vi "Durability_will_2012_07_04_motor not running.vi"() -> ()   [LabVIEW 2011]
uses:
  <vilib>/DAQmx/write.llb/DAQmx Write (Counter Time 1Chan 1Samp).vi
  <vilib>/DAQmx/read.llb/DAQmx Read (Analog 1D Wfm NChan NSamp).vi
  <vilib>/express/express shared/ex_Modify Signal Name.vi
  <vilib>/measure/madcrms.llb/Basic Averaged DC-RMS for 1 Chan.vi
  <vilib>/DAQmx/miscellaneous.llb/DAQmx Fill In Error Info.vi
  <vilib>/measure/madcrms.llb/Averaged DC-RMS for N Chan.vi
  <vilib>/express/express arith-compare/Formula/XNode/ExpressFormulaBlockNode.xnode
  <vilib>/measure/NI_MAPro.lvlib
panel:
  out "Collected Signals":dbl
  out "Table":string[][](table)
  in  "Filename 2":path=path "\\\\vmware-host\\Shared Folders/Desktop/long.tdms" caption="Filename"
  in  "Filename":path=path "\\\\vmware-host\\Shared Folders/Desktop/short.tdms"
  out "RPM Graph":dbl(graph)
  out "Motor RPM":dbl format="%#.0f"
  out "Motor Power (watts)":dbl format="%#.4f"
  out "Power to MC1 (watts)":dbl format="%#.4f"
  out "Voltage to MC1 (volts)":dbl format="%#.4f"
  out "Current to MC1  (amps)":dbl format="%#.4f"
  in  "Manual Start":bool
  in  "Power \nSetting":i8(slide) min=0 max=100 step=10 scale=0.0..100.0
  out "Power Setting (%)":dbl format="%#.2f"
  out "Motor Temp (F)":dbl format="%.1f"
  out "Tank Temp (F)":dbl format="%.1f"
  in  "Quit 4":bool
  out "Motor Power Over Time":dbl(graph)
  out "Phase to Phase Voltage":waveform(dbl)(graph)
  out "Phase Current":waveform(dbl)(graph)
  # "Motor Power and RPM"
  # "Temperature"
  # "MC1"
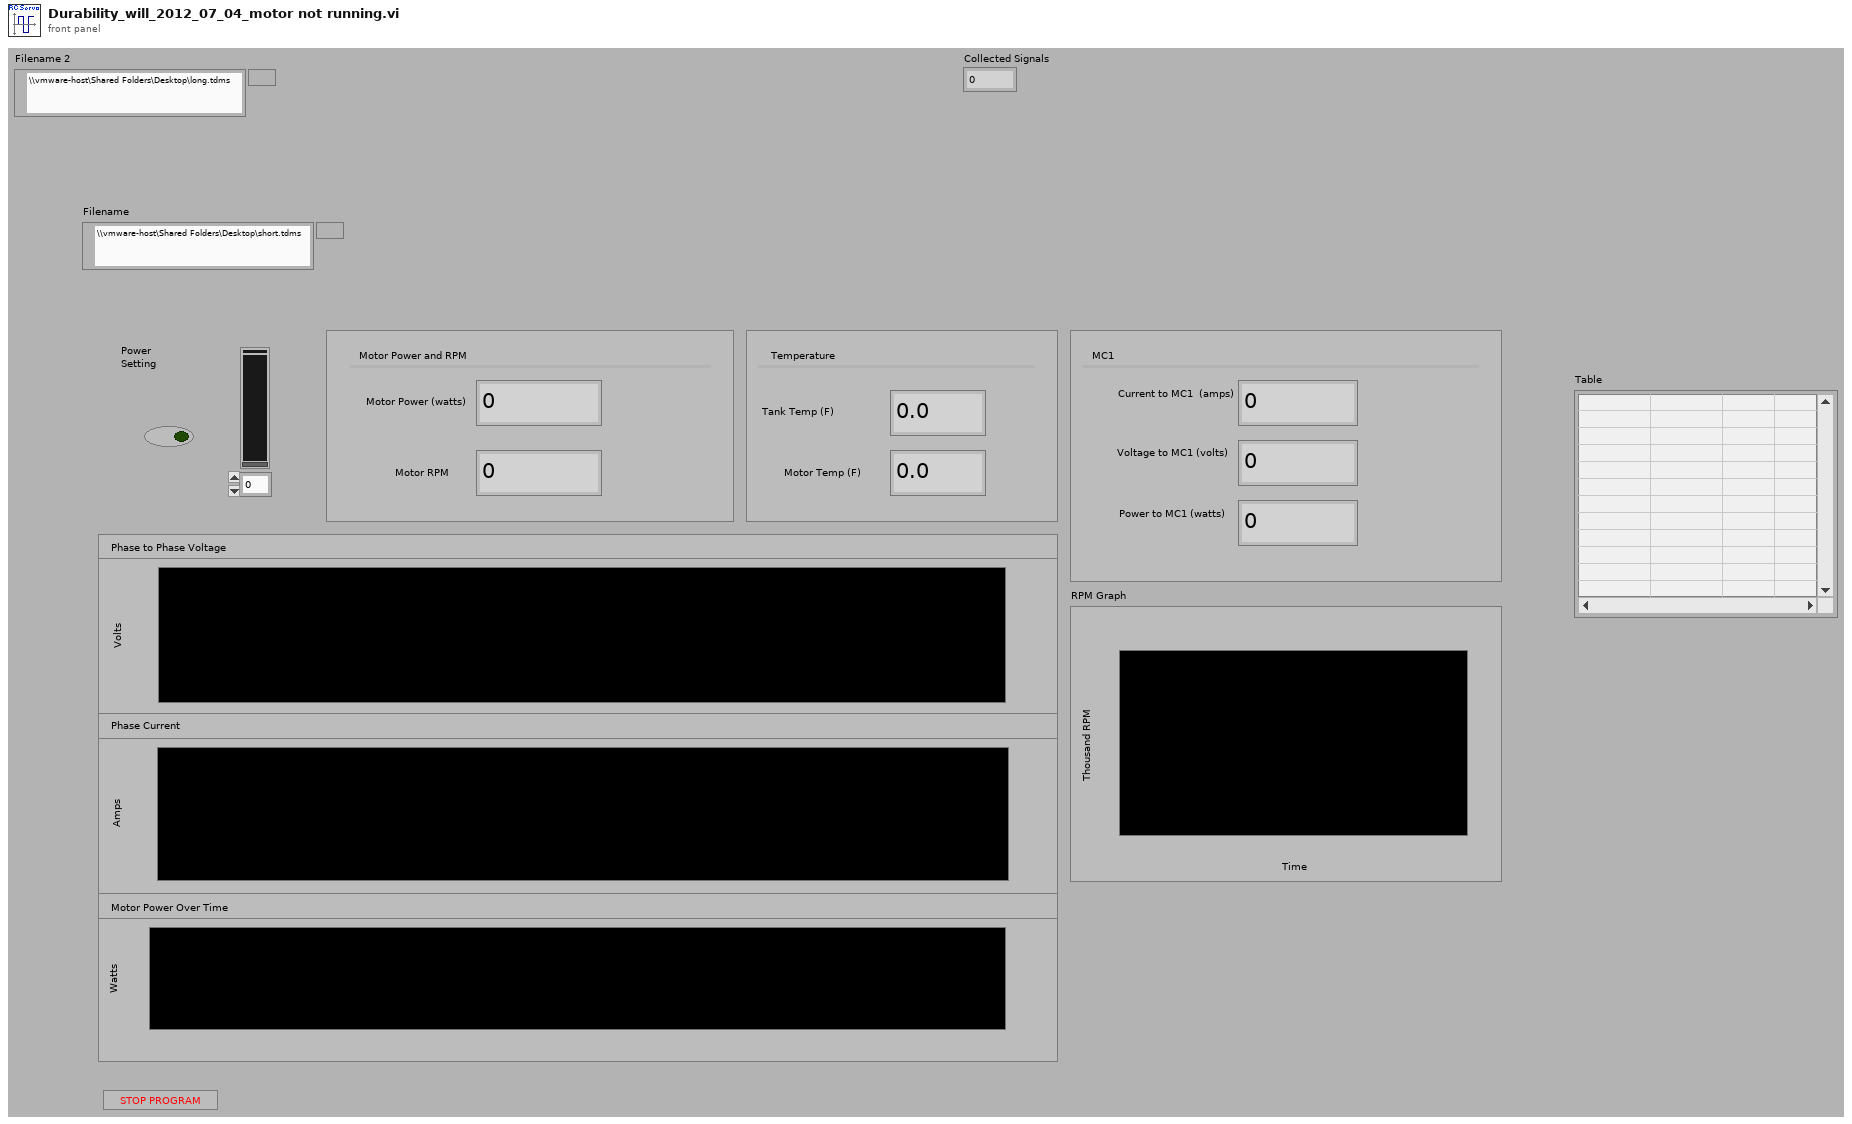
[diagram p1: front panel]
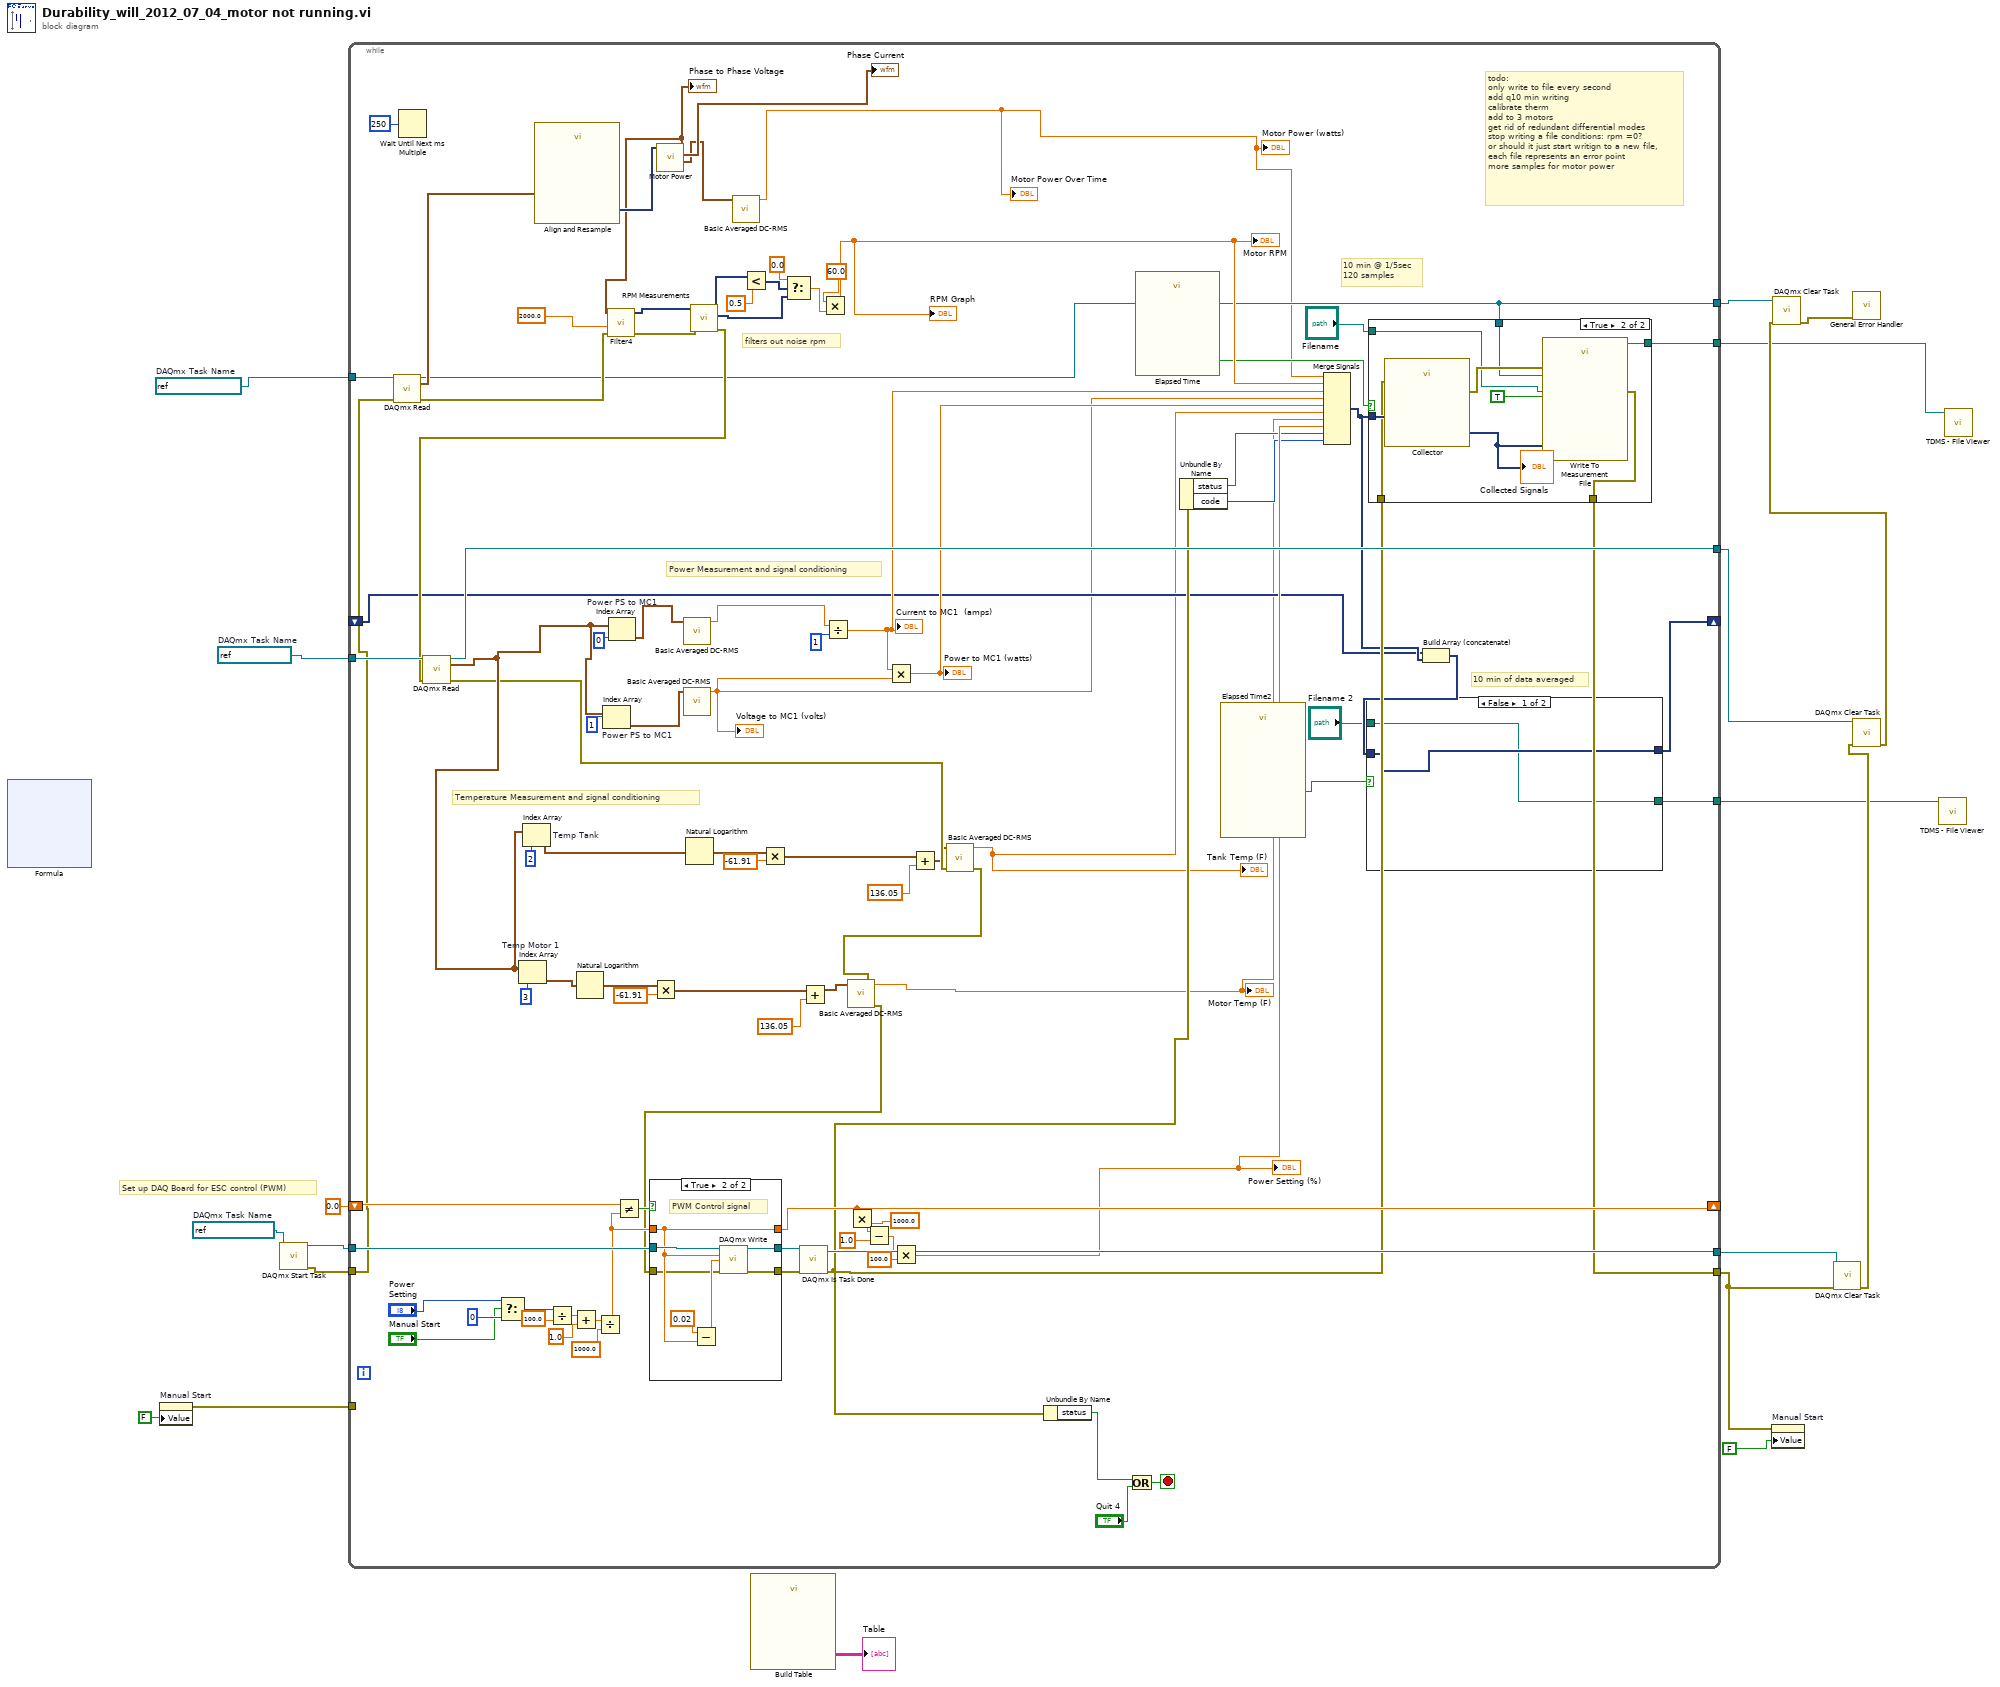
[diagram p0: block diagram]
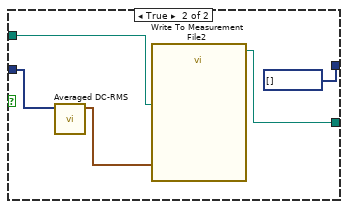
[diagram p2: hidden frame]
diagram:
  w10 = refnum<k21> "PWM Signal"  # DAQmx Task Name
  w15 = refnum<k21> "MC Power"  # DAQmx Task Name
  w16 = refnum<k21> "Motor Power"  # DAQmx Task Name
  # "Set up DAQ Board for ESC control (PWM)"
  n1 = xnode "Formula"() -> ()  [unwired: 2 in, 2 out]
  n2 = property on="Manual Start" class="Bool (strict)"("Value"=FALSE ("Run Motor")) -> (error out=w13:errorcluster)  [unwired: 2 in, 1 out]
  n3 = call <vilib>:"DAQmx Start Task.vi"("task/channels in"=w10) -> ("task out"=w9:refnum<k21>, "error out"=w8:errorcluster)  [unwired: 13 in]
  n4 = while {
    tunnel: [w113] -> w19
    tunnel: [w46] -> w11
    tunnel: w9 -> [w111]
    shift-right: [w94] -> _
    shift-left: 0.0 -> [w102]
    tunnel: w15 -> [w89]
    tunnel: [w88] -> w18
    tunnel: [w45] -> w17
    tunnel: w16 -> [w75]
    tunnel: w13 -> [_]
    tunnel: w8 -> [w68]
    shift-right: [w39] -> _
    shift-left: _ -> [w41]
    tunnel: [w38] -> w4
    tunnel: [w35] -> w3
    stop <- w71 stop-if-true
    # "10 min of data averaged"
    # "todo:\nonly write to file every second\nadd q10 min writing\ncalibrate therm\nadd to 3 motors\nget rid of redundant differential modes\nstop writing a file conditions: rpm =0?\nor should it just start writign to a new file,\neach file represents an error point\nmore samples for motor power"
    # "filters out noise rpm"
    # "10 min @ 1/5sec\n120 samples"
    # "Power Measurement and signal conditioning"
    # "Temperature Measurement and signal conditioning"
    n5 = call-poly <vilib>:"DAQmx Read.vi"("task/channels in"=w75, "error in"=w68) -> ("task out"=w45:refnum<k21>, "data"=w50:waveform(dbl)[], "error out"=w85:errorcluster)  [unwired: 11 in]
    n6 = Wait Until Next ms Multiple(millisecond multiple=u32 250) -> ()  [unwired: 1 out]
    n7 = Select(t="Power \nSetting", s="Manual Start", f=i8 0) -> (s? t:f=w100:i8)
    n8 = call "Align and Resample"("Signals"=w50) -> ("Resampled Signals"=w51:dynamicdata)  [unwired: 8 in, 2 out]
    n9 = Divide(x=w100, y=100.0) -> (x/y=w106:dbl)
    n10 = Add(x=w106, y=1.0 ("x/y")) -> (x+y=w104:dbl)
    n11 = Divide(x=w104, y=1000.0) -> (x/y=w103:dbl)
    n12 = Not Equal?(x=w102, y=w103) -> (x != y?=w112:bool)
    n13 = call "Motor Power.vi"("data"=w51) -> ("Waveform"=w34:waveform(dbl), "Phase Current"=→"Phase Current":waveform(dbl), "Phase to Phase Voltage"=w48:waveform(dbl))  [unwired: 7 in, 1 out]
    "Phase to Phase Voltage" <- w48
    n14 = call "Filter4"("error in (no error)"=w85, "Lower Cut-Off"=2000.0 ("LowPass Filter CutOff [Hz]"), "Signal"=w48) -> ("error out"=w86:errorcluster, "Filtered Signal"=w77:dynamicdata)  [unwired: 7 in]
    n15 = call "RPM Measurements"("error in (no error)"=w86, "Signals"=w77) -> ("error out"=w70:errorcluster, "Frequency"=w81:dynamicdata, "Amplitude"=w78:dynamicdata)  [unwired: 7 in]
    n16 = call-poly <vilib>:"DAQmx Read.vi"("task/channels in"=w89, "error in"=w70) -> ("task out"=w88:refnum<k21>, "data"=w27:waveform(dbl)[], "error out"=w25:errorcluster)  [unwired: 11 in]
    n17 = Index Array "Temp Motor 1"(array=w27, index=3) -> (element=w63:waveform(dbl))
    n18 = Index Array "Temp Tank"(array=w27, index=2) -> (element=w28:waveform(dbl))
    n19 = Natural Logarithm(1:w63) -> (0:w67:waveform(dbl))
    n20 = Index Array "Power PS to MC1"(array=w27, index=1) -> (element=w30:waveform(dbl))
    n21 = Index Array "Power PS to MC1"(array=w27, index=0) -> (element=w32:waveform(dbl))
    n22 = Multiply(x=w67, y=-61.91) -> (x*y=w65:waveform(dbl))
    n23 = call-poly <vilib>:"Basic Averaged DC-RMS.vi"("signal in"=w32) -> ("DC value"=w31:dbl)  [unwired: 7 in, 3 out]
    n24 = call-poly <vilib>:"Basic Averaged DC-RMS.vi"("signal in"=w30) -> ("DC value"=w29:dbl)  [unwired: 7 in, 3 out]
    "Voltage to MC1 (volts)" <- w29
    n25 = Natural Logarithm(1:w28) -> (0:w62:waveform(dbl))
    n26 = call-poly <vilib>:"Basic Averaged DC-RMS.vi"("signal in"=w34) -> ("DC value"=w33:dbl)  [unwired: 7 in, 3 out]
    "Motor Power Over Time" <- w33
    "Motor Power (watts)" <- w33
    n27 = Less?(x=w78, y=0.5) -> (x < y?=w80:dynamicdata)
    n28 = Multiply(x=w62, y=-61.91) -> (x*y=w60:waveform(dbl))
    n29 = Select(t=0.0, s=w80, f=w81) -> (s? t:f=w83:dbl)
    n30 = Add(x=w65, y=136.05) -> (x+y=w23:waveform(dbl))
    n31 = Multiply(x=60.0, y=w83) -> (x*y=w57:dbl)
    "Motor RPM" <- w57
    "RPM Graph" <- w57
    n32 = Divide(x=w31, y=1) -> (x/y=w56:dbl)
    "Current to MC1  (amps)" <- w56
    n33 = Multiply(x=w56, y=w29) -> (x*y=w55:dbl)
    "Power to MC1 (watts)" <- w55
    n34 = Add(x=w60, y=136.05) -> (x+y=w24:waveform(dbl))
    n35 = call-poly <vilib>:"Basic Averaged DC-RMS.vi"("error in (no error)"=w25, "signal in"=w24) -> ("error out"=w20:errorcluster, "DC value"=w26:dbl)  [unwired: 6 in, 2 out]
    "Tank Temp (F)" <- w26
    n36 = call-poly <vilib>:"Basic Averaged DC-RMS.vi"("error in (no error)"=w20, "signal in"=w23) -> ("error out"=w21:errorcluster, "DC value"=w22:dbl)  [unwired: 6 in, 2 out]
    "Motor Temp (F)" <- w22
    n37 = case shown="True" w112 {
      tunnel: w103 -> [w133 w136]
      tunnel: w111 -> [w134 w140]
      tunnel: [w134 w138] -> w110
      tunnel: [w132 w137] -> w109
      tunnel: [w133 w136] -> w94
      tunnel: w21 -> [w132 w135]
      frame False {
      }
      frame True {
        # "PWM Control signal"
        n38 = Subtract(x=0.02, y=w136) -> (x-y=w139:dbl)
        n39 = call-poly <vilib>:"DAQmx Write.vi"("task/channels in"=w140, "high time"=w136, "low time"=w139, "error in"=w135) -> ("task out"=w138:refnum<k21>, "error out"=w137:errorcluster)  [unwired: 9 in, 1 out]
      }
    }
    n40 = call <vilib>:"DAQmx Is Task Done.vi"("task/channels in"=w110, "error in"=w109) -> ("task out"=w113:refnum<k21>, "error out"=w47:errorcluster)  [unwired: 11 in, 1 out]
    n41 = Multiply(x=w94, y=1000.0) -> (x*y=w95:dbl)
    n42 = Subtract(x=w95, y=1.0) -> (x-y=w98:dbl)
    n43 = Multiply(x=w98, y=100.0) -> (x*y=w54:dbl)
    "Power Setting (%)" <- w54
    n44 = Unbundle By Name(w47) -> ("status"=w69:bool)
    n45 = Or(x=w69, y="Quit 4") -> (x .or. y?=w71:bool)
    n46 = call "Elapsed Time"() -> ("Time has Elapsed"=w44:bool)  [unwired: 12 in, 7 out]
    n47 = Unbundle By Name(w47) -> ("status"=w53:bool, "code"=w52:i32)
    n48 = call "Elapsed Time2"() -> ("Time has Elapsed"=w43:bool)  [unwired: 12 in, 7 out]
    n49 = Merge Signals(w33, w57, w56, w29, w55, w26, w22, w54, w53, w52) -> (w42:dynamicdata)
    n50 = case shown="True" w44 {
      tunnel: w42 -> [_ w131]
      tunnel: w47 -> [w122 w129]
      tunnel: [w122 w127] -> w46
      tunnel: w45 -> [_ w125]
      tunnel: "Filename" -> [w121 w124]
      tunnel: [w121 w123] -> w35
      frame False {
      }
      frame True {
        n51 = call "Collector"("error in (no error)"=w129, "Signals"=w131) -> ("error out"=w128:errorcluster, "Collected Signals"=w130:dynamicdata)  [unwired: 8 in]
        "Collected Signals" <- w130
        n52 = call "Write To Measurement File"("Signals"=w130, "Reset"=TRUE, "error in (no error)"=w128, "Filename"=w124, "DAQmx Task"=w125) -> ("Filename Out"=w123:path, "error out"=w127:errorcluster)  [unwired: 12 in, 1 out]
      }
    }
    n53 = Build Array (concatenate)(w41, w42) -> (w40:dynamicdata[])
    n54 = case shown="False" w43 {
      tunnel: w40 -> [w115 w119]
      tunnel: [w115 dynamicdata[] []] -> w39
      tunnel: [w114 w117] -> w38
      tunnel: "Filename 2" -> [w114 w116]
      frame False {
      }
      frame True {
        n55 = call-poly <vilib>:"Averaged DC-RMS.vi"("signals in"=w119) -> ("DC value waveforms"=w118:waveform(dbl)[])  [unwired: 6 in, 4 out]
        n56 = call "Write To Measurement File2"("Signals"=w118, "Filename"=w116) -> ("Filename Out"=w117:path)  [unwired: 15 in, 2 out]
      }
    }
  }
  n57 = call "Build Table"() -> ("Table"=→"Table":string[][])  [unwired: 5 in, 6 out]
  n58 = property on="Manual Start" class="Bool (strict)"(error in=w11, "Value"=FALSE ("Run Motor")) -> ()  [unwired: 1 in, 2 out]
  n59 = call <vilib>:"DAQmx Clear Task.vi"("task in"=w19, "error in"=w11) -> ("error out"=w5:errorcluster)  [unwired: 13 in]
  n60 = call <vilib>:"DAQmx Clear Task.vi"("task in"=w18, "error in"=w5) -> ("error out"=w7:errorcluster)  [unwired: 13 in]
  n61 = call <vilib>:"DAQmx Clear Task.vi"("task in"=w17, "error in"=w7) -> ("error out"=w6:errorcluster)  [unwired: 13 in]
  n62 = call <vilib>:"General Error Handler.vi"("error in (no error)"=w6) -> ()  [unwired: 10 in, 5 out]
  n63 = call <vilib>:"TDMS - File Viewer.vi"("file path"=w4) -> ()  [unwired: 1 in, 6 out]
  n64 = call <vilib>:"TDMS - File Viewer.vi"("file path"=w3) -> ()  [unwired: 1 in, 6 out]
